vi "API Constants.vi"() -> (3 "DAQmx IO Folder":string)   [LabVIEW 2021, in "Acquisition.lvlib"]
doc: "Return hard-coded values."
uses:
  Acquisition.lvlib
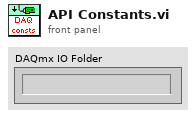
[diagram p1: front panel]
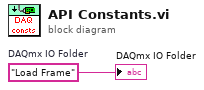
[diagram p0: block diagram]
diagram:
  w1 = "Load Frame"  # DAQmx IO Folder
  "DAQmx IO Folder" <- w1
